vi "test.vi"() -> ()   [LabVIEW 2023]
uses:
  vi.support/control/Parameters.ctl
panel:
  out "Waveform Graph":dbl[](graph)
  in  "line":i32
  out "XY Graph":cluster{"Z":i32[], "Param":dbl[]}[](graph)
  in  "Parameters Out":T1[](array[typedef])
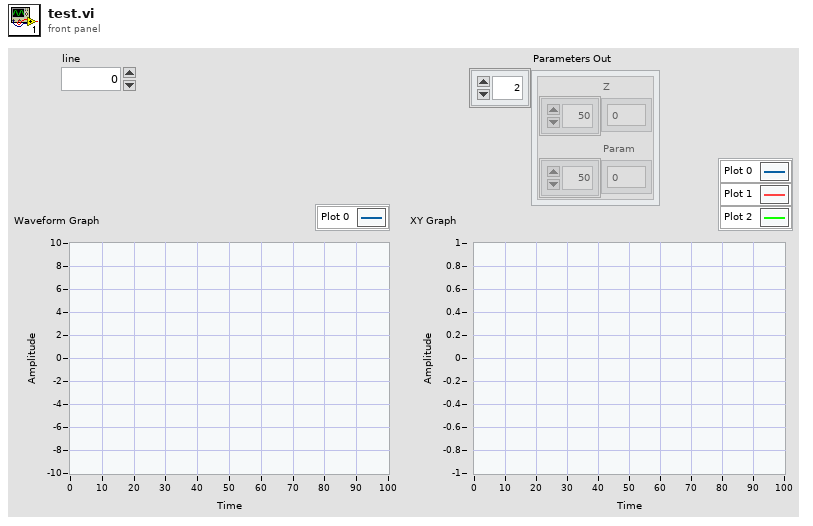
[diagram p1: front panel]
types:
  T1 = typedef "Parameters.ctl" = cluster{"Z":i32[], "Param":dbl[]}
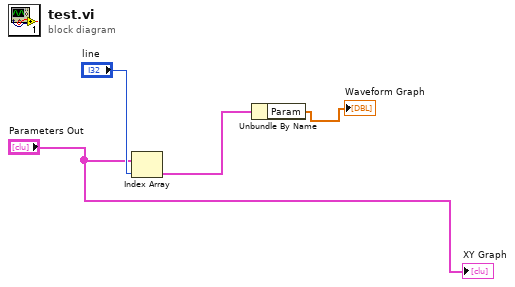
[diagram p0: block diagram]
diagram:
  n1 = Index Array(array="Parameters Out", index="line") -> (element=w2:T1)
  n2 = Unbundle By Name(w2) -> ("Param"=→"Waveform Graph":dbl[])
  "XY Graph" <- "Parameters Out"
